vi "dIMU_Gyro_rads.vi"(7 "Port":T2 items=["Port 1", "Port 2", "Port 3", "Port 4"], 9 "Gyro Scale":u8(ring)=16 items=["250 deg/s"=0, "500 deg/s"=16, "2000 deg/s"=32], 11 "NXT":T1={"Hardware"="NXT", "Flattened String"=""}) -> (0 "Z Gyro (rad/s":dbl, 1 "Y Gyro (rad/s)":dbl, 2 "X Gyro (rad/s)":dbl, 3 "NXT":T1={"Hardware"="NXT", "Flattened String"=""})   [LabVIEW 2010]
uses:
  <vilib>/NXT/Subs/LVHSConnector.ctl
  <vilib>/NXT/Block Support/NXT_InputPort.ctl
  <vilib>/NXT/Block Support/HWPage.SensorType.ctl
  <vilib>/NXT/Block Support/HWPage.SensorMode.ctl
  <vilib>/NXT/Dual Mode Library/Sensors/i2c_sensors.vi
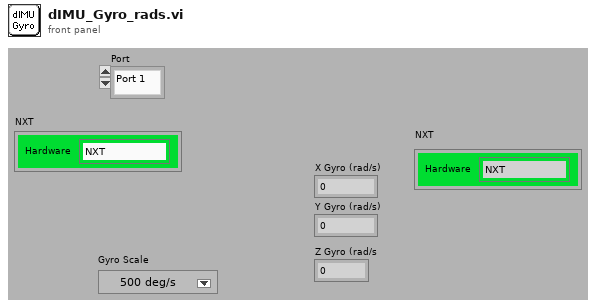
[diagram p1: front panel]
types:
  T1 = typedef "LVHSConnector.ctl" = cluster{"Hardware":string, "Flattened String":string}
  T2 = typedef "NXT_InputPort.ctl" = u8
  T3 = typedef "HWPage.SensorType.ctl" = u8
  T4 = typedef "HWPage.SensorMode.ctl" = u8
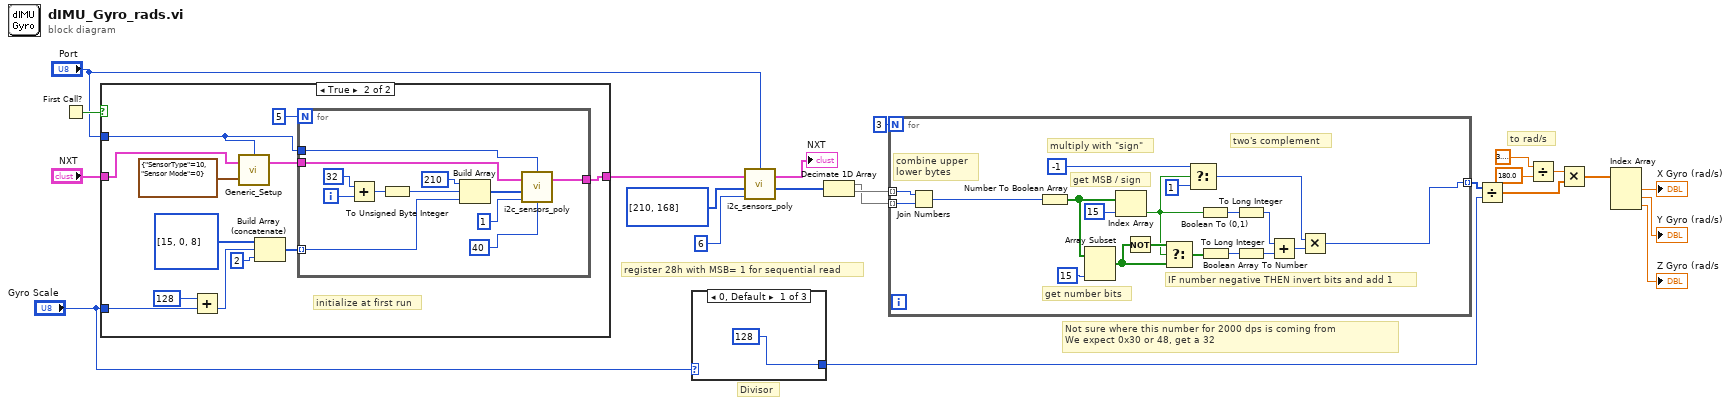
[diagram p0: block diagram]
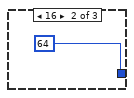
[diagram p2: hidden frame]
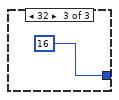
[diagram p3: hidden frame]
diagram:
  # "Not sure where this number for 2000 dps is coming from\nWe expect 0x30 or 48, get a 32"
  # "Divisor"
  # "to rad/s"
  # "register 28h with MSB= 1 for sequential read"
  n1 = First Call?() -> (First Call?: T/F=w22:bool)
  n2 = case shown="True" w22 {
    tunnel: [w23 w32] -> w18
    tunnel: "NXT" -> [w23 w31]
    tunnel: "Port" -> [_ w30]
    tunnel: "Gyro Scale" -> [_ w26]
    frame False {
    }
    frame True {
      # "initialize at first run"
      n3 = Add(x=u8 128, y=w26) -> (x+y=w25:u8)
      n4 = call <vilib>:"Generic_Setup.vi"("Sensor Setup"=cluster{"SensorType":T3, "Sensor Mode":T4} {"SensorType"=10, "Sensor Mode"=0}, "NXT"=w31, "Port"=w30) -> ("NXT"=w33:T1)  [unwired: 1 out]
      n5 = Build Array (concatenate)(u8[] [15, 0, 8], w25, u8 2 ("element")) -> (w27:u8[])
      n6 = for {
        N: 5 -> [_]
        tunnel: w33 -> [w47]
        tunnel: w30 -> [w46]
        tunnel: [w37] -> w32
        tunnel: w27 -> [w36] mode=indexing
        i -> [w44]
        n7 = Add(x=32, y=w44) -> (x+y=w42:i32)
        n8 = To Unsigned Byte Integer(number=w42) -> (unsigned 8bit integer=w41:u8)
        n9 = Build Array(u8 210, w41, w36) -> (w40:u8[])
        n10 = call-poly <vilib>:"i2c_sensors_poly.vi"("Return Length"=u8 1, "Bytes to Write"=w40, "Wait (msec)"=u32 40, "NXT"=w47, "Port"=w46) -> ("NXT"=w37:T1)  [unwired: 2 out]
      }
    }
  }
  n11 = case shown="0, Default" "Gyro Scale" {
    tunnel: [u8 128 ("f") u8 64 ("f") u8 16 ("f")] -> w3
    frame 0, Default {
    }
    frame 16 {
    }
    frame 32 {
    }
  }
  n12 = call-poly <vilib>:"i2c_sensors_poly.vi"("Return Length"=u8 6, "Bytes to Write"=u8[] [210, 168], "NXT"=w18, "Port"="Port") -> ("Bytes read"=w17:u8[], "NXT"=→"NXT":T1)  [unwired: 1 in, 1 out]
  n13 = Decimate 1D Array(w17) -> (w14:u8[], w15:u8[])
  n14 = for {
    N: 3 -> [_]
    tunnel: w15 -> [w69] mode=indexing
    tunnel: w14 -> [w68] mode=indexing
    tunnel: [w51] -> w4 mode=indexing
    # "two's complement"
    # "combine upper\nlower bytes"
    # "multiply with \"sign\""
    # "IF number negative THEN invert bits and add 1"
    # "get number bits"
    # "get MSB / sign"
    n15 = Join Numbers(hi=w69, lo=w68) -> ((hi.lo)=w52:u16)
    n16 = Number To Boolean Array(number=w52) -> (Boolean array=w53:bool[])
    n17 = Array Subset(array=w53, length=15) -> (w55:bool[])  [unwired: 1 in]
    n18 = Index Array(array=w53, index=15) -> (element=w56:bool)
    n19 = Not(x=w55) -> (.not. x?=w64:bool[])
    n20 = Select(t=w64, s=w56, f=w55) -> (s? t:f=w54:bool[])
    n21 = Select(t=-1, s=w56, f=1) -> (s? t:f=w59:i32)
    n22 = Boolean To (0,1)(Boolean=w56) -> (0, 1=w62:i16)
    n23 = Boolean Array To Number(Boolean array=w54) -> (number=w65:u32)
    n24 = To Long Integer(number=w62) -> (32bit integer=w57:i32)
    n25 = To Long Integer(number=w65) -> (32bit integer=w63:i32)
    n26 = Add(x=w57, y=w63) -> (x+y=w58:i32)
    n27 = Multiply(x=w59, y=w58) -> (x*y=w51:i32)
  }
  n28 = Divide(x=w4, y=w3) -> (x/y=w2:dbl[])
  n29 = Divide(x=3.141592653589793, y=180.0) -> (x/y=w6:dbl)
  n30 = Multiply(x=w6, y=w2) -> (x*y=w1:dbl[])
  n31 = Index Array(array=w1) -> (element #1=→"X Gyro (rad/s)":dbl, element #2=→"Y Gyro (rad/s)":dbl, element #3=→"Z Gyro (rad/s":dbl)  [unwired: 3 in]
